vi "Descriptor_ExtractElements.vi"(10 "Descriptor":T1) -> (0 "concatenated element descriptors":i16[](array[numeric]), 1 "Nb elements":i32, 2 "Descriptor Elements":T1[](array[typedef]))   [LabVIEW 2020, in "OpenDescriptor.lvlib"]
uses:
  OpenDescriptor.lvlib
  OpenDescriptor -- cluster.ctl
  TypeDescriptor_GetPString.vi
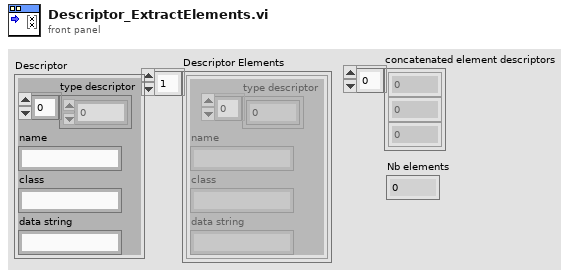
[diagram p1: front panel]
types:
  T1 = typedef "OpenDescriptor.lvlib/OpenDescriptor -- cluster.ctl" = cluster{"type descriptor":i16[], "name":string, "class":string, "data string":string}
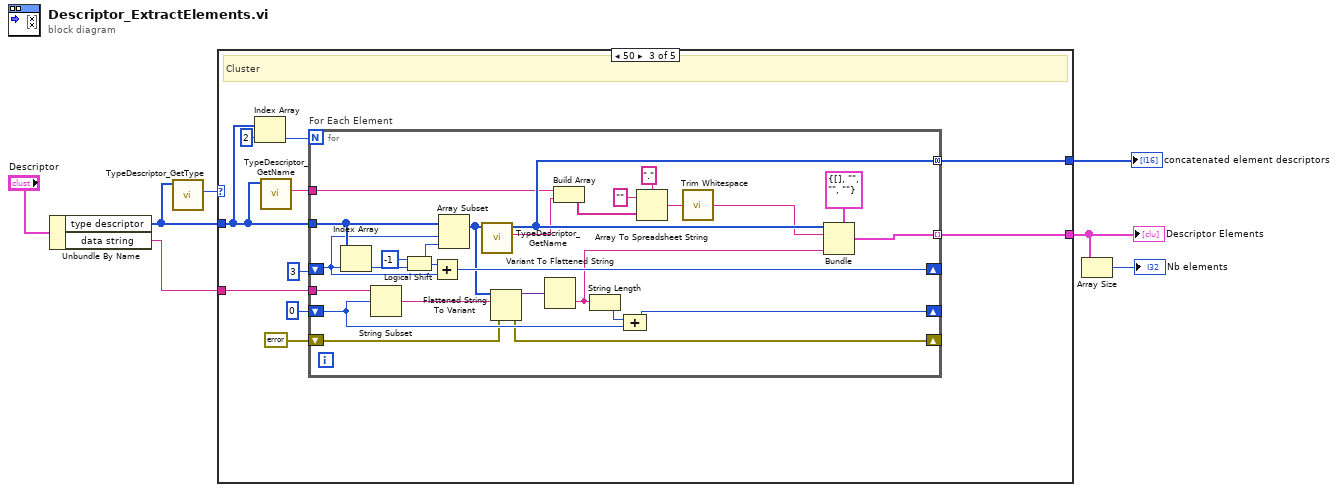
[diagram p0: block diagram]
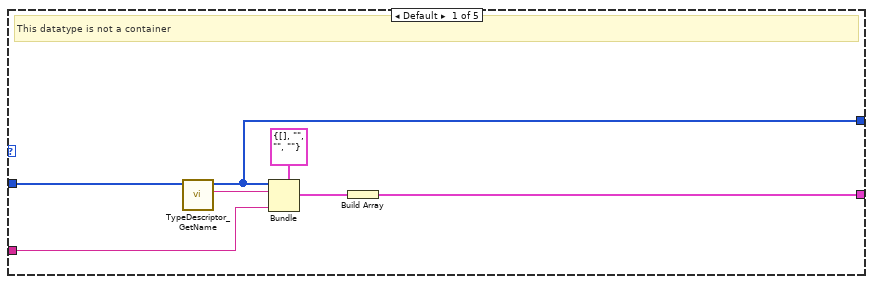
[diagram p2: hidden frame]
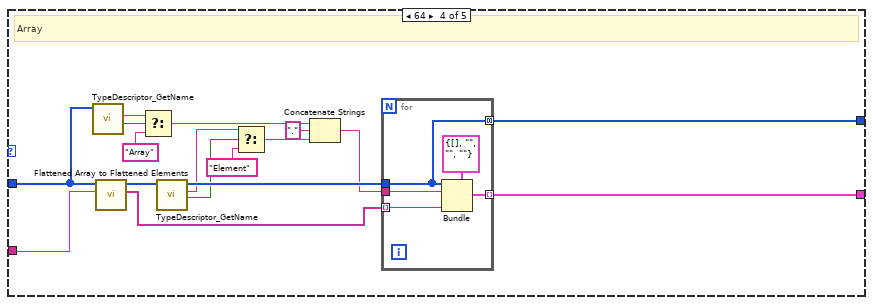
[diagram p4: hidden frame]
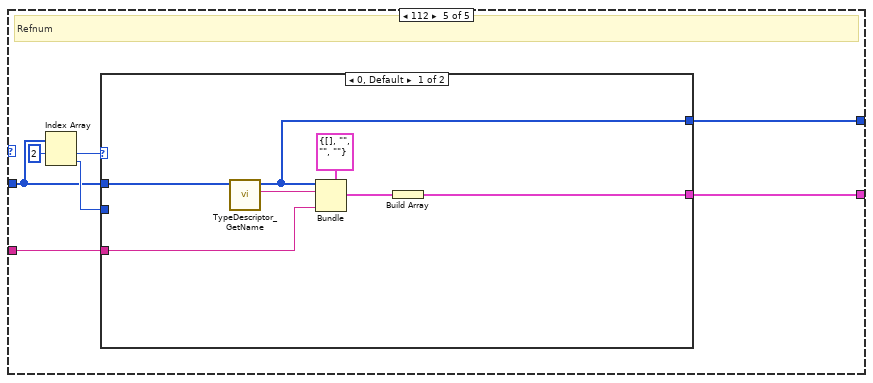
[diagram p5: hidden frame]
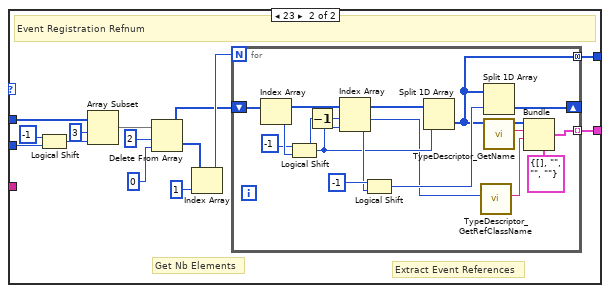
[diagram p6: hidden frame]
diagram:
  n1 = Unbundle By Name("Descriptor") -> ("type descriptor"=w2:i16[], "data string"=w1:string)
  n2 = call "TypeDescriptor_GetType.vi"("type descriptor"=w2) -> ("Type"=w3:u8)  [unwired: 9 in, 1 out]
  n3 = case shown="50" w3 {
    tunnel: [w10 _ w21 w64 w75] -> w7
    tunnel: w2 -> [w12 _ w16 w54 w76]
    tunnel: [w9 _ w20 w63 w74] -> w5
    tunnel: w1 -> [w8 _ w18 w53 w73]
    frame Default {
      # "This datatype is not a container"
      n4 = call "TypeDescriptor_GetName.vi"("type descriptor"=w12) -> ("name"=w14:string, "type descriptor dup"=w9:i16[])  [unwired: 8 in, 1 out]
      n5 = Bundle(cluster=T1 {"type descriptor"=[], "name"="", "class"="", "data string"=""} ("Descriptor Element"), "type descriptor"=w9, "name"=w14, "data string"=w8) -> (w11:T1)  [unwired: 1 in]
      n6 = Build Array(w11) -> (w10:T1[])
    }
    frame 0 {
      # "void"
    }
    frame 80 {
      # "Cluster"
      n7 = Index Array(array=w16, index=2) -> (element=w23:i16)
      n8 = call "TypeDescriptor_GetName.vi"("type descriptor"=w16) -> ("name"=w15:string)  [unwired: 8 in, 2 out]
      n9 = for "For Each Element" {
        N: w23 -> [_]
        tunnel: w16 -> [w47]
        shift-right: [w48] -> _
        shift-left: 3 ("index") -> [w46]
        tunnel: [w44] -> w21 mode=indexing
        tunnel: [w42] -> w20 mode=concatenating
        shift-right: [w35] -> _
        shift-left: 0 -> [w36]
        tunnel: w18 -> [w41]
        shift-right: [w32] -> _
        shift-left: errorcluster {"status"=FALSE, "code"=0, "source"=""} ("error out") -> [w33]
        tunnel: w15 -> [w31]
        n10 = Index Array(array=w47, index=w46) -> (element=w49:i16)
        n11 = String Subset(string=w41, offset (0)=w36) -> (substring=w39:string)  [unwired: 1 in]
        n12 = Logical Shift(y=i16 -1, x=w49) -> (x << y=w45:i16)
        n13 = Add(x=w45, y=w46) -> (x+y=w48:i32)
        n14 = Array Subset(array=w47, index=w46, length=w45) -> (w40:i16[])
        n15 = call "TypeDescriptor_GetName.vi"("type descriptor"=w40) -> ("name"=w30:string, "type descriptor dup"=w42:i16[])  [unwired: 8 in, 1 out]
        n16 = Flattened String To Variant(4:w33, 6:w39, 7:w40) -> (0:w32:errorcluster, 3:w38:variant)
        n17 = Variant To Flattened String(Variant=w38) -> (data string=w34:string)  [unwired: 1 out]
        n18 = Build Array(w31, w30) -> (w26:string[])
        n19 = String Length(string=w34) -> (length=w37:i32)
        n20 = Compound Arithmetic op=ADD(w37, w36) -> (w35:i32)
        n21 = Array To Spreadsheet String(delimiter (Tab)=".", array=w26, 3:"" ("format string")) -> (spreadsheet string=w29:string)
        n22 = call <vilib>:"Trim Whitespace.vi"("string"=w29) -> ("trimmed string"=w25:string)  [unwired: 1 in]
        n23 = Bundle(cluster=T1 {"type descriptor"=[], "name"="", "class"="", "data string"=""} ("Descriptor Element"), "type descriptor"=w42, "name"=w25, "data string"=w34) -> (w44:T1)  [unwired: 1 in]
      }
    }
    frame 64 {
      # "Array"
      n24 = call "TypeDescriptor_GetName.vi"("type descriptor"=w54) -> ("found"=w62:bool, "name"=w61:string)  [unwired: 8 in, 1 out]
      n25 = call "Flattened Array to Flattened Elements.vi"("Flattened Array String"=w53, "Array Type Descriptor"=w54) -> ("Flattened Array Elements"=w51:string[], "Array Element Type Descriptor"=w52:i16[])  [unwired: 8 in]
      n26 = Select(t=w61, s=w62, f="Array" ("string")) -> (s? t:f=w59:string)
      n27 = call "TypeDescriptor_GetName.vi"("type descriptor"=w52) -> ("found"=w55:bool, "name"=w56:string, "type descriptor dup"=w67:i16[])  [unwired: 8 in]
      n28 = Select(t=w56, s=w55, f="Element" ("string")) -> (s? t:f=w57:string)
      n29 = Concatenate Strings(w59, "." ("string"), w57) -> (w65:string)
      n30 = for {
        tunnel: w51 -> [w68] mode=indexing
        tunnel: [w71] -> w64 mode=indexing
        tunnel: w67 -> [w69]
        tunnel: w65 -> [w70]
        tunnel: [w69] -> w63 mode=concatenating
        n31 = Bundle(cluster=T1 {"type descriptor"=[], "name"="", "class"="", "data string"=""} ("Descriptor Element"), "type descriptor"=w69, "name"=w70, "data string"=w68) -> (w71:T1)  [unwired: 1 in]
      }
    }
    frame 112 {
      # "Refnum"
      n32 = Index Array(array=w76, index #1=2 ("index")) -> (element #1=w78:i16, element #2=w77:i16)  [unwired: 1 in]
      n33 = case shown="0, Default" w78 {
        tunnel: w77 -> [_ w97]
        tunnel: w76 -> [w83 w100]
        tunnel: [w81 w88] -> w75
        tunnel: [w82 w87] -> w74
        tunnel: w73 -> [w80 _]
        frame 0, Default {
          n34 = call "TypeDescriptor_GetName.vi"("type descriptor"=w83) -> ("name"=w84:string, "type descriptor dup"=w82:i16[])  [unwired: 8 in, 1 out]
          n35 = Bundle(cluster=T1 {"type descriptor"=[], "name"="", "class"="", "data string"=""} ("Descriptor Element"), "type descriptor"=w82, "name"=w84, "data string"=w80) -> (w86:T1)  [unwired: 1 in]
          n36 = Build Array(w86) -> (w81:T1[])
        }
        frame 23 {
          # "Extract Event References"
          # "Get Nb Elements"
          # "Event Registration Refnum"
          n37 = Logical Shift(y=i16 -1, x=w97) -> (x << y=w96:i16)
          n38 = Array Subset(array=w100, index=3, length=w96) -> (w95:i16[])
          n39 = Delete From Array(array=w95, length=2 ("index"), index=0) -> (deleted portion=w93:i16[], array with subset deleted=w89:i16[])
          n40 = Index Array(array=w93, index=1) -> (element=w90:i16)
          n41 = for {
            N: w90 -> [_]
            shift-right: [w108] -> _
            shift-left: w89 -> [w111]
            tunnel: [w103] -> w88 mode=indexing
            tunnel: [w101] -> w87 mode=concatenating
            n42 = Index Array(array=w111) -> (element=w116:i16)  [unwired: 1 in]
            n43 = Logical Shift(y=i16 -1, x=w116) -> (x << y=w110:i16)
            n44 = Decrement(x=w110) -> (x-1=w112:i16)
            n45 = Index Array(array=w111, index #1=w112, index #2=w110) -> (element #1=w107:i16, element #2=w113:i16)
            n46 = Logical Shift(y=i16 -1, x=w113) -> (x << y=w109:i16)
            n47 = Split 1D Array(array=w111, index=w110) -> (second subarray=w101:i16[])  [unwired: 1 out]
            n48 = call "TypeDescriptor_GetRefClassName.vi"("Ref Class"=w107) -> ("Reference Class"=w105:string)  [unwired: 10 in]
            n49 = Split 1D Array(array=w101, index=w109) -> (second subarray=w108:i16[])  [unwired: 1 out]
            n50 = call "TypeDescriptor_GetName.vi"("type descriptor"=w101) -> ("name"=w104:string, "type descriptor dup"=w106:i16[])  [unwired: 8 in, 1 out]
            n51 = Bundle(cluster=T1 {"type descriptor"=[], "name"="", "class"="", "data string"=""} ("Descriptor Element"), "type descriptor"=w106, "name"=w104, "class"=w105) -> (w103:T1)  [unwired: 1 in]
          }
        }
      }
    }
  }
  "Descriptor Elements" <- w7
  "concatenated element descriptors" <- w5
  n52 = Array Size(array=w7) -> (size(s)=→"Nb elements":i32)
